vi "Validate Plugin Name.vi"(0 "Name Input":string) -> (1 "Comparison Result":T1, 2 "Plugin Name":T2)   [LabVIEW 2015, in "Startup Processes.lvlib"]
uses:
  Startup Processes.lvlib
  _typedefs/Subpanel Names.ctl
  _typedefs/Name Valid Flag.ctl
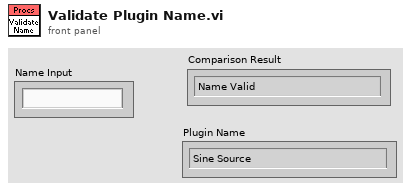
[diagram p1: front panel]
types:
  T1 = typedef "Startup Processes.lvlib/Name Valid Flag.ctl" = enum16{"Name Valid", "Name Not Valid"}
  T2 = typedef "Startup Processes.lvlib/Subpanel Names.ctl" = enum16{"Sine Source", "Ramp Source", "Hen House TC", "Dog House TC", "Out House TC"}
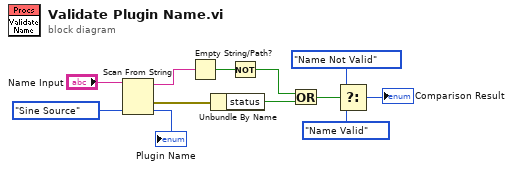
[diagram p0: block diagram]
diagram:
  n1 = Scan From String(input string="Name Input", default 1=Subpanel_Names."Sine Source" ("Plugin Names")) -> (remaining string=w5:string, error out=w6:errorcluster, output 1=→"Plugin Name":T2)  [unwired: 3 in, 1 out]
  n2 = Empty String/Path?(string/path=w5) -> (empty?=w2:bool)
  n3 = Unbundle By Name(w6) -> ("status"=w3:bool)
  n4 = Not(x=w2) -> (.not. x?=w1:bool)
  n5 = Or(x=w1, y=w3) -> (x .or. y?=w4:bool)
  n6 = Select(t=Name_Valid_Flag."Name Not Valid" ("Comparison Result"), s=w4, f=Name_Valid_Flag."Name Valid" ("Comparison Result")) -> (s? t:f=→"Comparison Result":T1)
